vi "State_Machine.vi"(8 "error in (no error)":errorcluster caption="entrée d'erreur (pas d'erreur)", 11 "Get_Voltage en entrée":refnum<class "Nodon_Get_HW_Version.lvclass">) -> (0 "error out":errorcluster caption="sortie d'erreur", 2 "Json_String":string, 3 "Get_Voltage en sortie":refnum<class "Nodon_Get_HW_Version.lvclass">)   [LabVIEW 2020, in "Library Test.lvlib" / "Nodon_Get_HW_Version.lvclass"]
uses:
  Nodon_Get_HW_Version.lvclass
  C:/Users/ngarcin/OneDrive - Altyor/Standard TB/Class/Test/Nodon_Send_Command_UART/Nodon_Send_Command_UART.lvclass
  Nodon_Send_Command_UART.lvclass
  Nodon_Get_HW_Version.lvclass/Nodon_Get_HW_Version.ctl
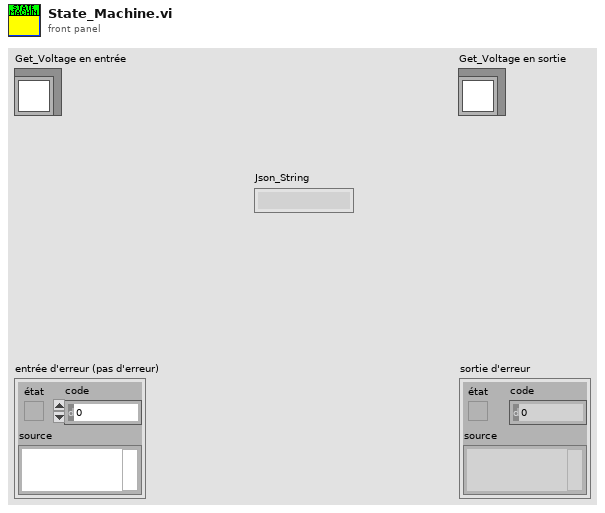
[diagram p1: front panel]
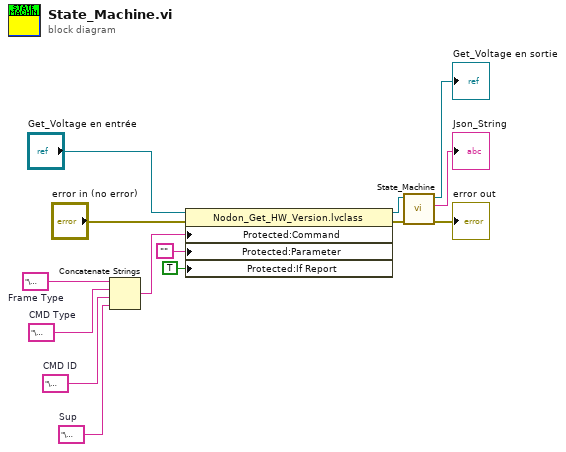
[diagram p0: block diagram]
diagram:
  w2 = "\u0001"  # Sup
  w6 = "\u0000"  # Frame Type
  w5 = "\u0000"  # CMD ID
  w4 = "\u0002"  # CMD Type
  n1 = Concatenate Strings(w6, w4, w5, w2) -> (w3:string)
  n2 = property class="Nodon_Get_HW_Version.lvclass"(reference="Get_Voltage en entrée", error in="error in (no error)", "Protected:Command"=w3, "Protected:Parameter"="", "Protected:If Report"=TRUE ("If Report")) -> (reference out=w9:refnum<class "Nodon_Get_HW_Version.lvclass">, error out=w7:errorcluster)
  n3 = call-parent "State_Machine.vi"("error in (no error)"=w7, "Send_Frame en entrée"=w9) -> ("error out"=→"error out":errorcluster, "Json_String"=→"Json_String":string, "Send_Frame en sortie"=→"Get_Voltage en sortie":refnum<class "Nodon_Get_HW_Version.lvclass">)  [unwired: 7 in]
